vi "Test.vi"   [LabVIEW 2016]
doc: "This VI is called when test mode begins, and will automatically be terminated when it ends. You can add manual or automatic tests and invoke them from the dashboard."
uses:
  <vilib>/Rock Robotics/Network Tables/NT Read Number.vi
types:
  T1 = typedef "WPI_MotorControlDeviceRef.ctl" = cluster{"DeviceStatus":errorcluster, "Type":T2, "PWM":cluster{"PWM Channel":T3, "DeadBand":T4}, "CAN":cluster{"Device Number":u8, "SetOutput VI Ref":variant, "GetOutput VI Ref":variant, "Enable VI Ref":variant, "Disable VI Ref":variant, "Data":variant}, "Invert":bool}
  T2 = typedef "WPI_MotorControlType.ctl" = enum16{"PWM", "CAN"}
  T3 = typedef "FPGA_DIOPWMChannel.ctl" = enum8{"PWM 0", "PWM 1", "PWM 2", "PWM 3", "PWM 4", "PWM 5", "PWM 6", "PWM 7", "PWM 8", "PWM 9", "PWM MXP 0", "PWM MXP 1", "PWM MXP 2", "PWM MXP 3", "PWM MXP 4", "PWM MXP 5", "PWM MXP 6", "PWM MXP 7", "PWM MXP 8", "PWM MXP 9", "Invalid"}
  T4 = typedef "WPI_PWMDeadband.ctl" = cluster{"Name":string, "maxPositivePwm":i32, "minPositivePwm":i32, "centerPwm":i32, "maxNegativePwm":i32, "minNegativePwm":i32, "angularRange":u16}
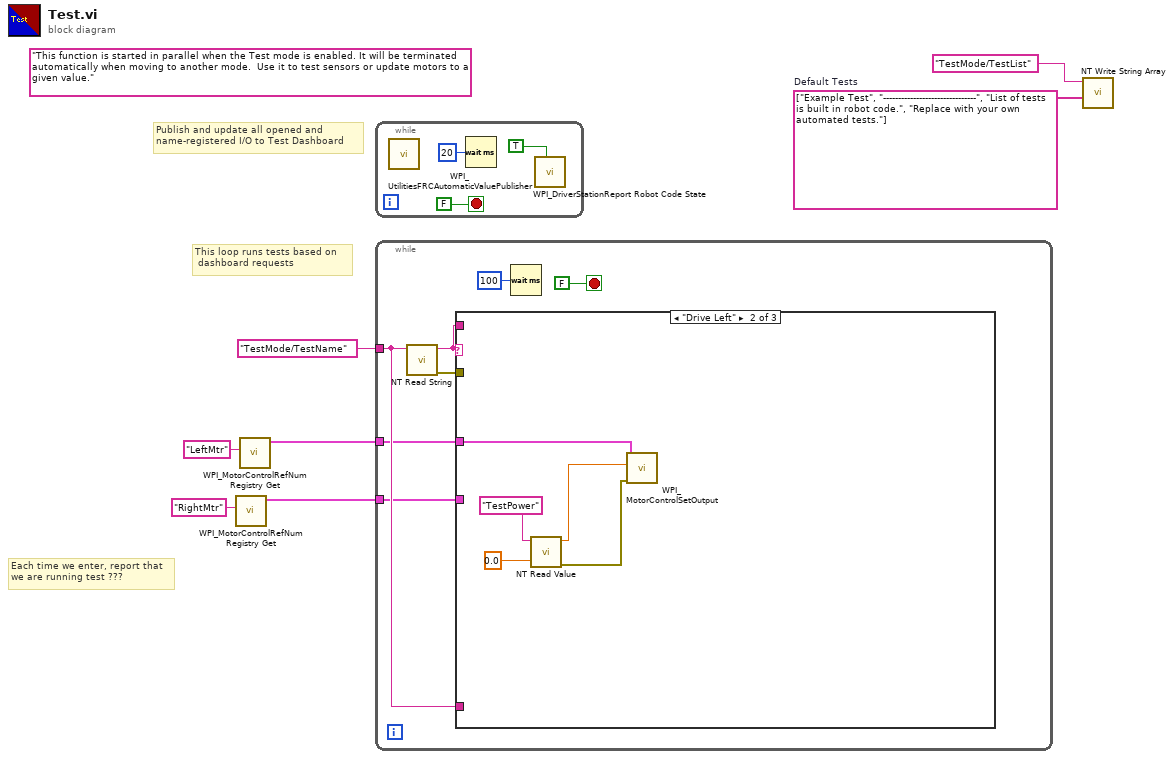
[diagram p0: block diagram]
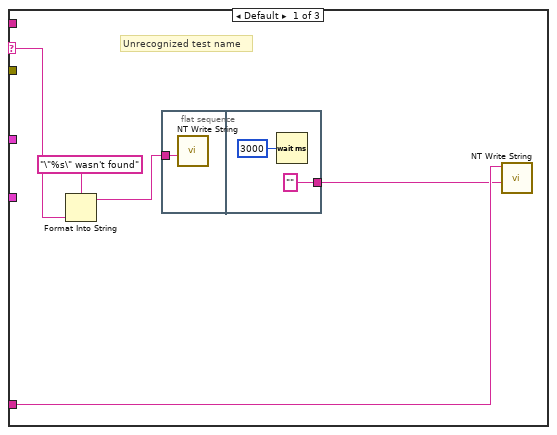
[diagram p2: hidden frame]
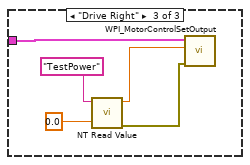
[diagram p3: hidden frame]
diagram:
  w6 = string[] ["Example Test", "-------------------------------", "List of tests is built in robot code.", "Replace with your own automated tests."]  # Default Tests
  (unwired) "This function is started in parallel when the Test mode is enabled. It will be terminated automatically when moving to another mode.  Use it to test sensors or update motors to a given value."
  # "This loop runs tests based on \n dashboard requests"
  # "Publish and update all opened and\nname-registered I/O to Test Dashboard"
  # "Each time we enter, report that\nwe are running test ???"
  n1 = call <vilib>:"WPI_MotorControlRefNum Registry Get.vi"("refnum name"="RightMtr") -> ("MotorControlDevRef"=w2:T1)  [unwired: 9 in, 1 out]
  n2 = call <vilib>:"WPI_MotorControlRefNum Registry Get.vi"("refnum name"="LeftMtr") -> ("MotorControlDevRef"=w1:T1)  [unwired: 9 in, 1 out]
  n3 = while {
    stop <- FALSE stop-if-true
    n4 = call <vilib>:"WPI_UtilitiesFRCAutomaticValuePublisher.vi"() -> ()  [unwired: 12 in]
    n5 = Wait (ms)(milliseconds to wait=u32 20) -> ()  [unwired: 1 out]
    n6 = call <vilib>:"WPI_DriverStationReport Robot Code State.vi"("Test"=TRUE ("Autonomous")) -> ()  [unwired: 10 in, 1 out]
  }
  n7 = while {
    tunnel: "TestMode/TestName" ("Name") -> [w14]
    tunnel: w2 -> [w12]
    tunnel: w1 -> [w11]
    stop <- FALSE stop-if-true
    n8 = call <vilib>:"NT Read String.vi"("Name"=w14) -> ("error out"=w13:errorcluster, "String"=w15:string)  [unwired: 9 in]
    n9 = case shown="\"Drive Left\"" w15 {
      selector: w15 -> [w22 _ _]
      tunnel: w14 -> [w19 _ _]
      tunnel: w15 -> [_ _ _]
      tunnel: w13 -> [_ _ _]
      tunnel: w12 -> [_ _ w35]
      tunnel: w11 -> [_ w30 _]
      frame Default {
        # "Unrecognized test name"
        n10 = Format Into String(format string="\"%s\" wasn't found" ("Name"), w22) -> (resulting string=w21:string)  [unwired: 2 in, 1 out]
        n11 = flat-sequence {
          tunnel: w21 -> [w23]
          tunnel: ["" ("Name")] -> w18
          frame #0 {
            n12 = call <vilib>:"NT Write String.vi"("String"=w23) -> ()  [unwired: 10 in, 1 out]
          }
          frame #1 {
            n13 = Wait (ms)(milliseconds to wait=u32 3000) -> ()  [unwired: 1 out]
          }
        }
        n14 = call <vilib>:"NT Write String.vi"("String"=w18, "Name"=w19) -> ()  [unwired: 9 in, 1 out]
      }
      frame "Drive Left" {
        n15 = call-poly <vilib>:"NT Read Value.vi"("Default Value"=0.0, "Name"="TestPower") -> ("error out"=w26:errorcluster, "Numeric"=w29:dbl)  [unwired: 8 in]
        n16 = call <vilib>:"WPI_MotorControlSetOutput.vi"("error in (no error)"=w26, "Output"=w29, "MotorControlDevRef"=w30) -> ()  [unwired: 6 in, 3 out]
      }
      frame "Drive Right" {
        n17 = call-poly <vilib>:"NT Read Value.vi"("Default Value"=0.0, "Name"="TestPower") -> ("error out"=w31:errorcluster, "Numeric"=w32:dbl)  [unwired: 8 in]
        n18 = call <vilib>:"WPI_MotorControlSetOutput.vi"("error in (no error)"=w31, "Output"=w32, "MotorControlDevRef"=w35) -> ()  [unwired: 6 in, 3 out]
      }
    }
    n19 = Wait (ms)(milliseconds to wait=u32 100) -> ()  [unwired: 1 out]
  }
  n20 = call <vilib>:"NT Write String Array.vi"("String Array"=w6, "Name"="TestMode/TestList") -> ()  [unwired: 9 in, 1 out]
